vi "Read Database.vi"(8 "error in":errorcluster, 10 "Suppress dialog?":bool, 11 "Path":path=path "C:/Users/Public/Documents/National Instruments/NI-XNET/Examples/NIXNET_example.xml") -> (0 "error out":errorcluster, 2 "Database":T1[](array[typedef]))   [LabVIEW 2020, in "Communication Bus Template System Explorer.lvlib" / "Implementation.lvlib"]
uses:
  Implementation.lvlib
  Types/Database.ctl
  Types/Frame.ctl
  Types/Signal.ctl
  Types/ECU.ctl
  Scripting/Constants.vi
  <resource>/objmgr/xnet.rc
  Scripting/Communication Bus Template Scripting.lvlib
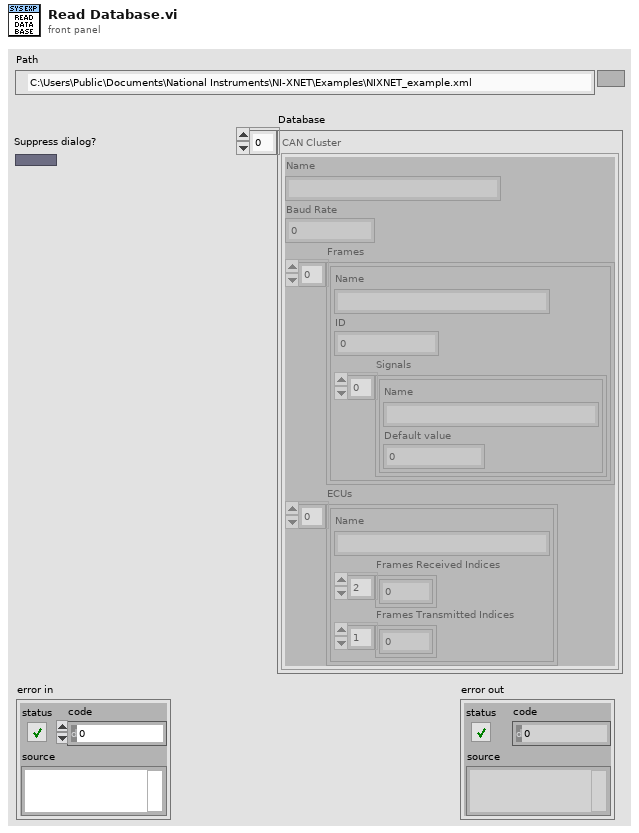
[diagram p1: front panel]
types:
  T1 = typedef "Communication Bus Template System Explorer.lvlib/Implementation.lvlib/Database.ctl" = cluster{"Name":string, "Baud Rate":u64, "Frames":T2[], "ECUs":T4[]}
  T2 = typedef "Communication Bus Template System Explorer.lvlib/Implementation.lvlib/Frame.ctl" = cluster{"Name":string, "ID":u32, "Signals":T3[]}
  T3 = typedef "Communication Bus Template System Explorer.lvlib/Implementation.lvlib/Signal.ctl" = cluster{"Name":string, "Default value":dbl}
  T4 = typedef "Communication Bus Template System Explorer.lvlib/Implementation.lvlib/ECU.ctl" = cluster{"Name":string, "Frames Received Indices":u32[], "Frames Transmitted Indices":u32[]}
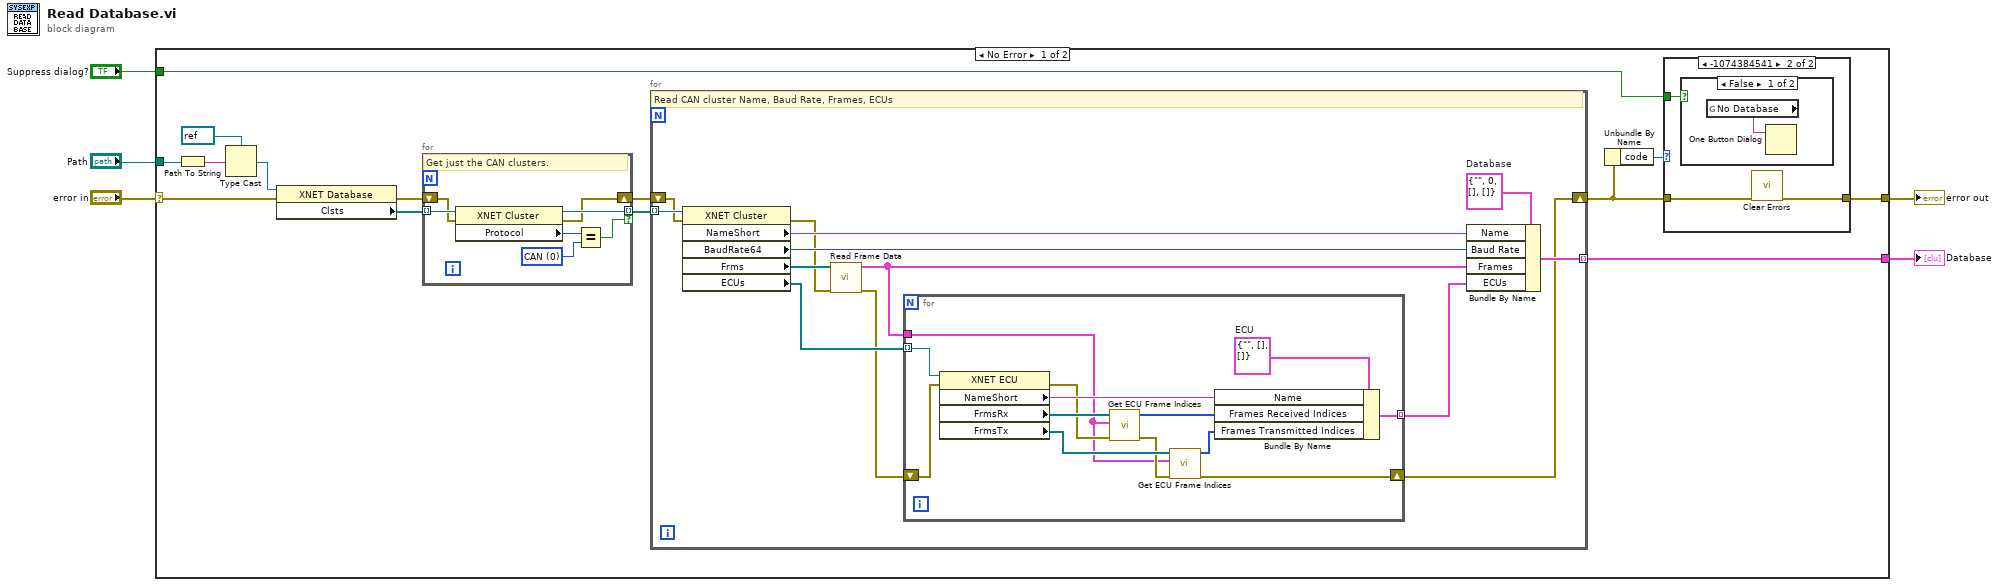
[diagram p0: block diagram]
diagram:
  n1 = case shown="No Error" "error in" {
    selector: "error in" -> [w15 w58]
    tunnel: "Path" -> [w16 _]
    tunnel: [w7 w58] -> w2
    tunnel: [w12 _] -> w3
    tunnel: "Suppress dialog?" -> [w6 _]
    frame No Error {
      n2 = Path To String(path=w16) -> (string=w17:string)
      n3 = Type Cast(type=refnum<k21> refnum ("XNET Database"), x=w17) -> (*(type *) &x=w19:refnum<k21>)
      n4 = property class="XNET Database"(reference=w19, error in=w15) -> (error out=w11:errorcluster, "Clsts"=w14:refnum<k21>[])  [unwired: 1 out]
      n5 = for {
        tunnel: w14 -> [w57] mode=indexing
        tunnel: [w56] -> w13 mode=indexing if=w54
        shift-right: [w51] -> w10
        shift-left: w11 -> [w52]
        w53 = u32 0 items=["CAN", "FlexRay", "LIN"] ("Protocol")
        # "Get just the CAN clusters."
        n6 = property class="XNET Cluster"(reference=w57, error in=w52) -> (reference out=w56:refnum<k21>, error out=w51:errorcluster, "Protocol"=w55:u32)
        n7 = Equal?(x=w55, y=w53) -> (x = y?=w54:bool)
      }
      n8 = for {
        tunnel: w13 -> [w37] mode=indexing
        shift-right: [w26] -> w8
        shift-left: w10 -> [w36]
        tunnel: [w34] -> w12 mode=indexing
        w33 = T1 {"Name"="", "Baud Rate"=0, "Frames"=[], "ECUs"=[]}  # Database
        # "Read CAN cluster Name, Baud Rate, Frames, ECUs"
        n9 = property class="XNET Cluster"(reference=w37, error in=w36) -> (error out=w30:errorcluster, "NameShort"=w32:string, "BaudRate64"=w35:u64, "Frms"=w31:refnum<k21>[], "ECUs"=w29:refnum<k21>[])  [unwired: 1 out]
        n10 = call "Read Frame Data.vi"("error in"=w30, "XNET Frames"=w31) -> ("error out"=w28:errorcluster, "Frames"=w25:T2[])  [unwired: 8 in]
        n11 = for {
          tunnel: w29 -> [w50] mode=indexing
          shift-right: [w39] -> w26
          shift-left: w28 -> [w49]
          tunnel: [w40] -> w27 mode=indexing
          tunnel: w25 -> [w38]
          w48 = T4 {"Name"="", "Frames Received Indices"=[], "Frames Transmitted Indices"=[]}  # ECU
          n12 = property class="XNET ECU"(reference=w50, error in=w49) -> (error out=w45:errorcluster, "NameShort"=w47:string, "FrmsRx"=w46:refnum<k21>[], "FrmsTx"=w44:refnum<k21>[])  [unwired: 1 out]
          n13 = call "Get ECU Frame Indices.vi"("error in"=w45, "Frames"=w38, "XNET Frames"=w46) -> ("error out"=w43:errorcluster, "Frame Indices"=w42:u32[])  [unwired: 7 in]
          n14 = call "Get ECU Frame Indices.vi"("error in"=w43, "Frames"=w38, "XNET Frames"=w44) -> ("error out"=w39:errorcluster, "Frame Indices"=w41:u32[])  [unwired: 7 in]
          n15 = Bundle By Name(cluster=w48, "Name"=w47, "Frames Received Indices"=w42, "Frames Transmitted Indices"=w41) -> (w40:T4)
        }
        n16 = Bundle By Name(cluster=w33, "Name"=w32, "Baud Rate"=w35, "Frames"=w25, "ECUs"=w27) -> (w34:T1)
      }
      n17 = Unbundle By Name(w8) -> ("code"=w9:i32)
      n18 = case shown="-1074384541" w9 {
        tunnel: [w20 w22] -> w7
        tunnel: w8 -> [w20 w23]
        tunnel: w6 -> [_ w21]
        frame Default {
        }
        frame -1074384541 {
          n19 = case shown="False" w21 {
            frame False {
              n20 = global read "Constants.vi" "No Database"() -> (w24:string)
              n21 = One Button Dialog(message=w24) -> ()  [unwired: 1 in, 1 out]
            }
            frame True {
            }
          }
          n22 = call <vilib>:"Clear Errors.vi"("error in (no error)"=w23) -> ("error out"=w22:errorcluster)  [unwired: 5 in, 1 out]
        }
      }
    }
    frame Error {
    }
  }
  "error out" <- w2
  "Database" <- w3
